vi "Write N Bytes.vi"(0 "COM Port":refnum<visa-resource-name>, 1 "Sector":i32 format="%x", 2 "NFC ID(ASCII)":string, 5 "Starting Page Address":i32 format="%x", 7 "Offset(Byte, 0-3)":i32 max=16 step=1, 9 "Data to Write (Hex)":string, 11 "Data to Write (ASCII)":string, 12 "Data in ASCII":bool, 13 "Reverse":bool) -> (4 "PN532 COM Port out":refnum<visa-resource-name>, 6 "Succeeded":bool, 15 "error out":errorcluster)   [LabVIEW 2012, in "NFC Driver.lvlib"]
uses:
  NFC Driver.lvlib
  <vilib>/Utility/error.llb/Error Cluster From Error Code.vi
  <vilib>/ErrorRing/Error Ring.xnode
panel:
  out "String":string
  out "concatenated string":string
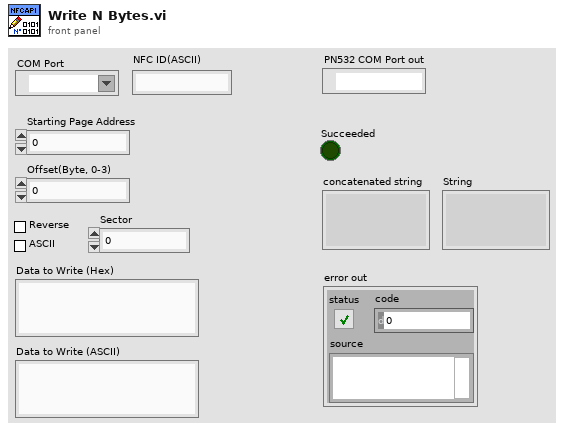
[diagram p1: front panel]
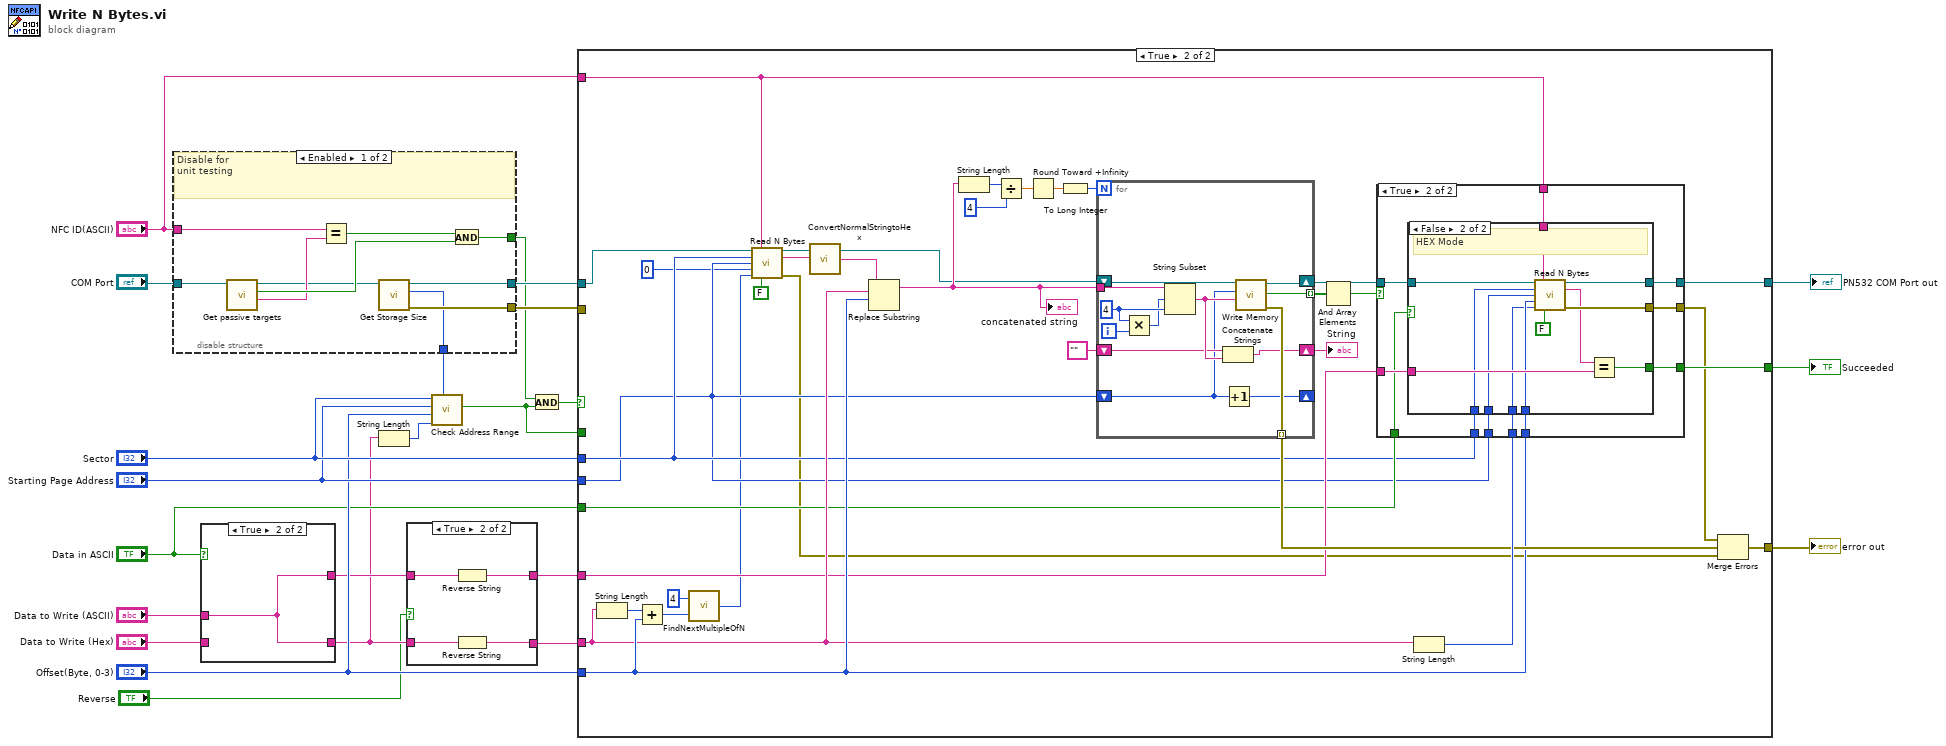
[diagram p0: block diagram]
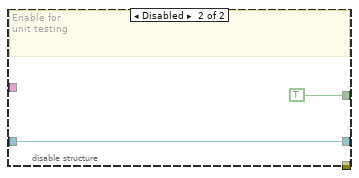
[diagram p3: hidden frame]
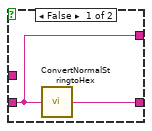
[diagram p4: hidden frame]
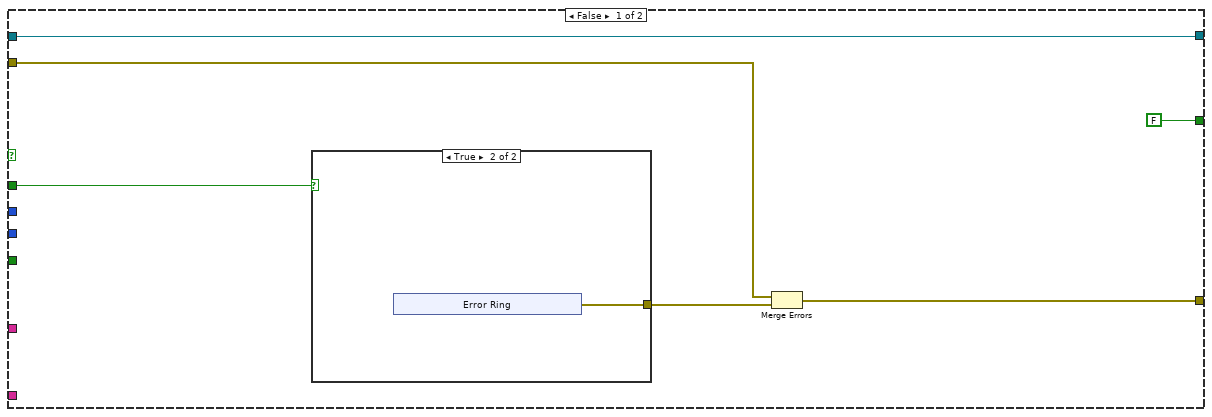
[diagram p5: hidden frame]
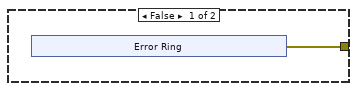
[diagram p6: hidden frame]
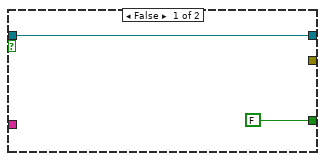
[diagram p7: hidden frame]
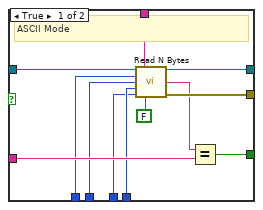
[diagram p8: hidden frame]
diagram:
  n1 = disable-structure shown="Enabled" {
    disable-tunnel: [w31 TRUE] -> w13
    disable-tunnel: "COM Port" -> [w28 w34]
    disable-tunnel: [w26 w34] -> w22
    disable-tunnel: [w25 _] -> w21
    disable-tunnel: "NFC ID(ASCII)" -> [w29 _]
    disable-tunnel: [w24 _] -> w11
    frame Enabled {
      # "Disable for\nunit testing"
      n2 = call "Get passive targets.vi"("PN532 COM Port"=w28) -> ("NFC ID (ASCII)"=w30:string, "Found?"=w32:bool, "PN532 COM Port Out"=w27:refnum<visa-resource-name>)  [unwired: 6 in, 2 out]
      n3 = Equal?(x=w29, y=w30) -> (x = y?=w33:bool)
      n4 = call "Get Storage Size.vi"("PN532 COM Port"=w27) -> ("error out"=w25:errorcluster, "Storage Size"=w24:i32, "PN532 COM Port out"=w26:refnum<visa-resource-name>)  [unwired: 8 in]
      n5 = And(x=w33, y=w32) -> (x .and. y?=w31:bool)
    }
    frame Disabled {
      # "Enable for \nunit testing"
    }
  }
  n6 = case shown="True" "Data in ASCII" {
    tunnel: [w37 w38] -> w3
    tunnel: "Data to Write (Hex)" -> [w36 _]
    tunnel: [w36 w38] -> w5
    tunnel: "Data to Write (ASCII)" -> [_ w38]
    frame False {
      n7 = call "ConvertNormalStringtoHex.vi"("Normal String"=w36) -> ("Hex String"=w37:string)
    }
    frame True {
    }
  }
  n8 = String Length(string=w3) -> (length=w15:i32)
  n9 = case shown="True" "Reverse" {
    tunnel: w5 -> [w40 w44]
    tunnel: [w40 w42] -> w4
    tunnel: [w39 w41] -> w2
    tunnel: w3 -> [w39 w43]
    frame False {
    }
    frame True {
      n10 = Reverse String(1:w44) -> (0:w42:string)
      n11 = Reverse String(1:w43) -> (0:w41:string)
    }
  }
  n12 = call "Check Address Range.vi"("Storage Size"=w11, "Length(Byte)"=w15, "Offset"="Offset(Byte, 0-3)", "Page(hex)"="Starting Page Address", "Sector"="Sector") -> ("Address In Range"=w7:bool)  [unwired: 6 in]
  n13 = And(x=w13, y=w7) -> (x .and. y?=w12:bool)
  n14 = case shown="True" w12 {
    tunnel: w22 -> [w45 w73]
    tunnel: w21 -> [w50 _]
    tunnel: "Starting Page Address" -> [_ w71]
    tunnel: w2 -> [_ w79]
    tunnel: "Offset(Byte, 0-3)" -> [_ w80]
    tunnel: [w48 w92] -> w20
    tunnel: "NFC ID(ASCII)" -> [_ w67]
    tunnel: [FALSE w95] -> w18
    tunnel: "Sector" -> [_ w72]
    tunnel: w4 -> [_ w77]
    tunnel: "Data in ASCII" -> [_ w76]
    tunnel: w7 -> [w46 _]
    tunnel: [w45 w74] -> w6
    frame False {
      n15 = case shown="True" w46 {
        tunnel: [w51 w57] -> w49
        frame False {
          n16 = xnode "Error Ring"() -> ("error out"=w51:errorcluster)
        }
        frame True {
          n17 = xnode "Error Ring"() -> ("error out"=w57:errorcluster)
        }
      }
      n18 = Merge Errors(w50, w49) -> (w48:errorcluster)
    }
    frame True {
      n19 = String Length(string=w79) -> (length=w83:i32)
      n20 = Add(x=w83, y=w80) -> (x+y=w82:i32)
      n21 = call "FindNextMultipleOfN.vi"("Input"=w82, "n"=4) -> ("Integer"=w69:i32)
      n22 = call "Read N Bytes.vi"("COM Port"=w73, "NFC ID(ASCII)"=w67, "Sector"=w72, "Starting Page Address"=w71, "Offset(0-3, Byte)"=0, "Length(Byte)"=w69, "Reverse Output[F]"=FALSE) -> ("PN532 COM Port out"=w66:refnum<visa-resource-name>, "Data(Hex)"=w65:string, "error out"=w64:errorcluster)  [unwired: 5 in, 1 out]
      n23 = call "ConvertNormalStringtoHex.vi"("Normal String"=w65) -> ("Hex String"=w63:string)
      n24 = Replace Substring(3:w80, 4:w79, 5:w63) -> (1:w78:string)  [unwired: 1 in, 1 out]
      "concatenated string" <- w78
      n25 = String Length(string=w78) -> (length=w90:i32)
      n26 = Divide(x=w90, y=4) -> (x/y=w88:dbl)
      n27 = Round Toward +Infinity(x=w88) -> (ceil(x): smallest int >= x=w87:dbl)
      n28 = To Long Integer(number=w87) -> (32bit integer=w86:i32)
      n29 = for {
        N: w86 -> [_]
        tunnel: w78 -> [w108]
        tunnel: [w99] -> w96 mode=indexing
        tunnel: [w109] -> w93 mode=indexing
        shift-right: [w102] -> w84
        shift-left: "" -> [w103]
        shift-right: [w100] -> _
        shift-left: w71 -> [w101]
        shift-right: [w98] -> w75
        shift-left: w66 -> [w110]
        i -> [w107]
        w106 = 4 ("length (rest)")
        n30 = Multiply(x=w106, y=w107) -> (x*y=w105:i32)
        n31 = String Subset(string=w108, offset (0)=w105, length (rest)=w106) -> (substring=w104:string)
        n32 = Concatenate Strings(w103, w104) -> (w102:string)
        n33 = Increment(x=w101) -> (x+1=w100:i32)
        n34 = call "Write Memory.vi"("Data to write (HEX, max 16 bytes)"=w104, "Page Address"=w101, "PN532 COM Port"=w110) -> ("Error Out"=w109:errorcluster, "Succesful?"=w99:bool, "PN532 COM Port Out"=w98:refnum<visa-resource-name>)  [unwired: 6 in]
      }
      "String" <- w84
      n35 = And Array Elements(Boolean array=w96) -> (logical AND=w91:bool)
      n36 = String Length(string=w79) -> (length=w97:i32)
      n37 = case shown="True" w91 {
        tunnel: w75 -> [w111 w120]
        tunnel: w71 -> [_ w118]
        tunnel: w97 -> [_ w116]
        tunnel: w80 -> [_ w117]
        tunnel: w67 -> [_ w121]
        tunnel: w77 -> [_ w123]
        tunnel: [FALSE w122] -> w95
        tunnel: [_ w115] -> w94
        tunnel: w72 -> [_ w119]
        tunnel: w76 -> [_ w114]
        tunnel: [w111 w113] -> w74
        frame False {
        }
        frame True {
          n38 = case shown="False" w114 {
            tunnel: w123 -> [w135 w147]
            tunnel: [w134 w146] -> w122
            tunnel: w121 -> [w133 w145]
            tunnel: w120 -> [w132 w144]
            tunnel: w119 -> [w130 w142]
            tunnel: w118 -> [w129 w141]
            tunnel: w117 -> [w128 w140]
            tunnel: w116 -> [w127 w139]
            tunnel: [w126 w138] -> w115
            tunnel: [w125 w136] -> w113
            frame True {
              # "ASCII Mode"
              n39 = call "Read N Bytes.vi"("COM Port"=w132, "NFC ID(ASCII)"=w133, "Sector"=w130, "Starting Page Address"=w129, "Offset(0-3, Byte)"=w128, "Length(Byte)"=w127, "Reverse Output[F]"=FALSE) -> ("PN532 COM Port out"=w125:refnum<visa-resource-name>, "Data(ASCII)"=w124:string, "error out"=w126:errorcluster)  [unwired: 5 in, 1 out]
              n40 = Equal?(x=w124, y=w135) -> (x = y?=w134:bool)
            }
            frame False {
              # "HEX Mode"
              n41 = call "Read N Bytes.vi"("COM Port"=w144, "NFC ID(ASCII)"=w145, "Sector"=w142, "Starting Page Address"=w141, "Offset(0-3, Byte)"=w140, "Length(Byte)"=w139, "Reverse Output[F]"=FALSE) -> ("PN532 COM Port out"=w136:refnum<visa-resource-name>, "Data(Hex)"=w137:string, "error out"=w138:errorcluster)  [unwired: 5 in, 1 out]
              n42 = Equal?(x=w137, y=w147) -> (x = y?=w146:bool)
            }
          }
        }
      }
      n43 = Merge Errors(w94, w93, w64) -> (w92:errorcluster)
    }
  }
  "error out" <- w20
  "Succeeded" <- w18
  "PN532 COM Port out" <- w6
